vi "Serial_Parser.vi"(11 "Trame":string) -> (0 "CRC":i32, 1 "PIR":i32, 2 "RPM":i32, 3 "STATE":string, 4 "Trame valide":bool)   [LabVIEW 2022 SP3]
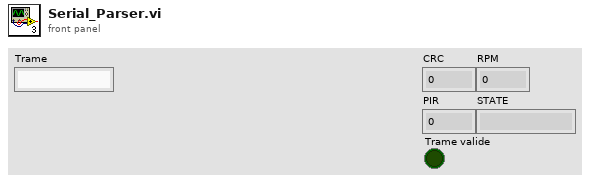
[diagram p1: front panel]
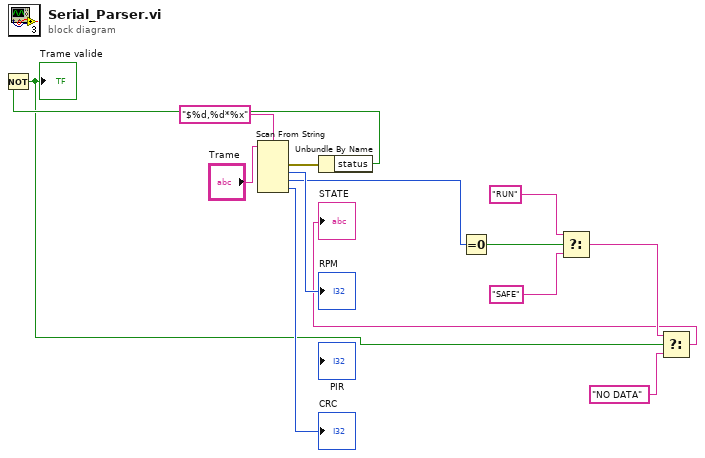
[diagram p0: block diagram]
diagram:
  n1 = Scan From String(format string="$%d,%d*%x", input string="Trame") -> (error out=w13:errorcluster, output 1=→"RPM":i32, output 2=w9:i32, output 3=→"CRC":i32)  [unwired: 5 in, 2 out]
  n2 = Unbundle By Name(w13) -> ("status"=w12:bool)
  n3 = Not(x=w12) -> (.not. x?=w2:bool)
  "Trame valide" <- w2
  n4 = Equal To 0?(x=w9) -> (x = 0?=w8:bool)
  n5 = Select(t="RUN", s=w8, f="SAFE") -> (s? t:f=w4:string)
  n6 = Select(t=w4, s=w2, f="NO DATA") -> (s? t:f=→"STATE":string)
